vi "WPI_PWMClose.vi"(8 "error in (no error)":errorcluster, 11 "PWMDeviceRef":T1={"DeviceStatus"={"status"=FALSE, "code"=0, "source"=""}, "PWM Channel"=enum."PWM 4"}) -> (0 "error out":errorcluster)   [LabVIEW 2017]
doc: "Closes the reference to the PWM or motor controller you specify. Use this VI to close each PWM reference that you open with the Open VI.\n\nThis software is licensed. Open the labview\\readme\\WPI Robotics Library Open Source License.txt file for more information."
uses:
  <vilib>/Rock Robotics/WPI/PWM/WPI_PWMDeviceRef.ctl
  <vilib>/Rock Robotics/SystemInterfaces/DIO/FPGA_DIOPWMChannel.ctl
  <vilib>/Rock Robotics/WPI/PWM/WPI_PWMChannelCacheOp.ctl
  <instrlib>/Parallax Standard Servo/HAIOL/Parallax Standard Servo.lvclass
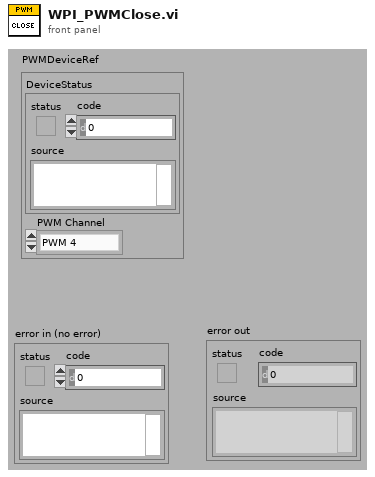
[diagram p1: front panel]
types:
  T1 = typedef "WPI_PWMDeviceRef.ctl" = cluster{"DeviceStatus":errorcluster, "PWM Channel":T2}
  T2 = typedef "FPGA_DIOPWMChannel.ctl" = enum8{"PWM 0", "PWM 1", "PWM 2", "PWM 3", "PWM 4", "PWM 5", "PWM 6", "PWM 7", "PWM 8", "PWM 9", "PWM MXP 0", "PWM MXP 1", "PWM MXP 2", "PWM MXP 3", "PWM MXP 4", "PWM MXP 5", "PWM MXP 6", "PWM MXP 7", "PWM MXP 8", "PWM MXP 9", "Invalid"}
  T3 = typedef "WPI_PWMChannelCacheOp.ctl" = enum16{"Acquire", "Release", "Status"}
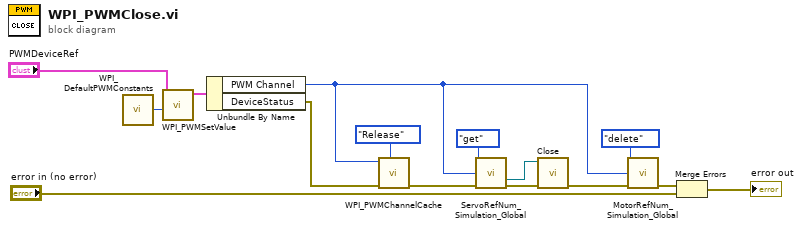
[diagram p0: block diagram]
diagram:
  n1 = call <vilib>:"WPI_DefaultPWMConstants.vi"() -> ("defaultPWMDisabled"=w12:u16)  [unwired: 1 in, 18 out]
  n2 = call <vilib>:"WPI_PWMSetValue.vi"("Value"=w12, "PWMDeviceRef"="PWMDeviceRef") -> ("PWMDeviceRef"=w11:T1)  [unwired: 2 in, 7 out]
  n3 = Unbundle By Name(w11) -> ("PWM Channel"=w1:T2, "DeviceStatus"=w14:errorcluster)
  n4 = call <vilib>:"WPI_PWMChannelCache.vi"("Operation"=WPI_PWMChannelCacheOp."Release", "error in (no error)"=w14, "PWMChannel"=w1) -> ("error out"=w2:errorcluster)  [unwired: 2 in, 6 out]
  n5 = call <vilib>:"ServoRefNum_Simulation_Global.vi"("menu"=enum16{"set", "get", "delete"}."get", "PWM Channel"=w1, "error in (no error)"=w2) -> ("Servo Get"=w6:refnum<class "Parallax Standard Servo.lvclass">, "error out"=w5:errorcluster)  [unwired: 11 in]
  n6 = call-dynamic "Close.vi"("error in (no error)"=w5, "Parallax Standard Servo in"=w6) -> ("error out"=w8:errorcluster)  [unwired: 9 in]
  n7 = call <vilib>:"MotorRefNum_Simulation_Global.vi"("menu"=enum16{"set", "get", "delete"}."delete", "PWM Channel"=w1, "error in (no error)"=w8) -> ("error out"=w3:errorcluster)  [unwired: 11 in, 1 out]
  n8 = Merge Errors(w3, "error in (no error)") -> (→"error out":errorcluster)
